vi "Verify and Check-in.vi"(0 "Rooms Manager Model in":refnum<class "Rooms Manager Model.lvclass">, 5 "Room No":string, 7 "Guest Contact Number":string, 9 "Primary Guest Name":string, 11 "error in (no error)":errorcluster, 12 "Adults":u32, 13 "Children":u32) -> (4 "Rooms Manager Model out":refnum<class "Rooms Manager Model.lvclass">, 15 "error out":errorcluster)   [LabVIEW 2023, in "Rooms Manager Model.lvlib" / "Rooms Manager Model.lvclass"]
uses:
  Rooms Manager Model.lvclass
  Rooms Manager Model.lvclass/Rooms Manager Model.ctl
  <vilib>/ActorFramework/Actor/Actor.lvclass
  Interfaces/Incoming Hotel Management Tool Model Interface Messages/Verify and Check-in Msg/Verify and Check-in Msg.lvclass
  C:/Users/bhaghyaraj/Trainings/NI Actor Framework/SDLC/Model Base/Model Base/Model Base.lvclass
  C:/Program Files/National Instruments/LabVIEW 2023/vi.lib/ActorFramework/Actor/Actor.lvclass
  C:/Users/bhaghyaraj/Trainings/NI Actor Framework/SDLC/Interfaces/Model Base/Incoming Model Base Interface.lvclass
  C:/Users/bhaghyaraj/Trainings/NI Actor Framework/SDLC/Rooms Manager Model/Rooms Manager Model/Rooms Manager Model.lvclass
  C:/Users/bhaghyaraj/Trainings/NI Actor Framework/SDLC/Interfaces/Rooms Manager Model/Incoming Rooms Manager Model Interface.lvclass
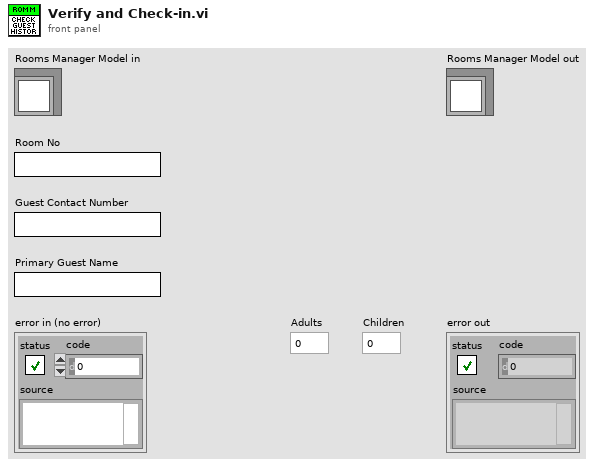
[diagram p1: front panel]
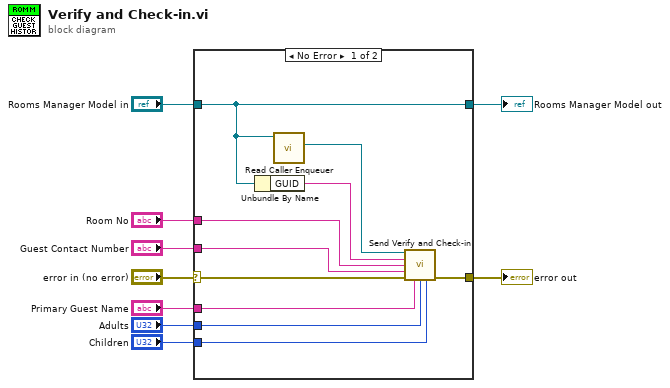
[diagram p0: block diagram]
diagram:
  n1 = case shown="No Error" "error in (no error)" {
    selector: "error in (no error)" -> [w17 w20]
    tunnel: [w18 w20] -> w6
    tunnel: "Rooms Manager Model in" -> [w19 w21]
    tunnel: [w19 w21] -> w8
    tunnel: "Room No" -> [w11 _]
    tunnel: "Guest Contact Number" -> [w10 _]
    tunnel: "Primary Guest Name" -> [w14 _]
    tunnel: "Adults" -> [w13 _]
    tunnel: "Children" -> [w12 _]
    frame No Error {
      n2 = Unbundle By Name(w19) -> ("GUID"=w15:string)
      n3 = call <vilib>:"Read Caller Enqueuer.vi"("Actor"=w19) -> ("Caller Enqueuer"=w16:refnum<class "Message Enqueuer.lvclass">)  [unwired: 10 in]
      n4 = call "Send Verify and Check-in.vi"("Message Enqueuer"=w16, "Rooms Manager GUID"=w15, "Room No"=w11, "Guest Contact Number In"=w10, "error in (no error)"=w17, "Primary Guest Name"=w14, "Adults"=w13, "Children"=w12) -> ("error out"=w18:errorcluster)  [unwired: 6 in, 1 out]
    }
    frame Error {
    }
  }
  "error out" <- w6
  "Rooms Manager Model out" <- w8
